vi "PXI-Create Channels.vi"(0 "Task Specification Array In":T1[](array[typedef]) {"Channels"."Terminal configuration" items=["Default"=-1, "RSE"=10083, "Differential"=10106, "Pseudodifferential"=12529]}, 11 "error in (no error)":errorcluster) -> (4 "Task Specification Array Out":T1[](array[typedef]) {"Channels"."Terminal configuration" items=["Default"=-1, "RSE"=10083, "Differential"=10106, "Pseudodifferential"=12529]}, 15 "error out":errorcluster)   [LabVIEW 2020]
uses:
  Type Defs/Task Specification Struct.ctl
  Type Defs/Channel Struct.ctl
  PXI Globals.vi
  <vilib>/DAQmx/create/channels.llb/DAQmx Create Channel (AI-Voltage-Basic).vi
  <vilib>/DAQmx/configure/timing.llb/DAQmx Timing (Sample Clock).vi
  <vilib>/DAQmx/create/channels.llb/DAQmx Create Channel (AO-Voltage-Basic).vi
  <resource>/objmgr/daqmx.rc
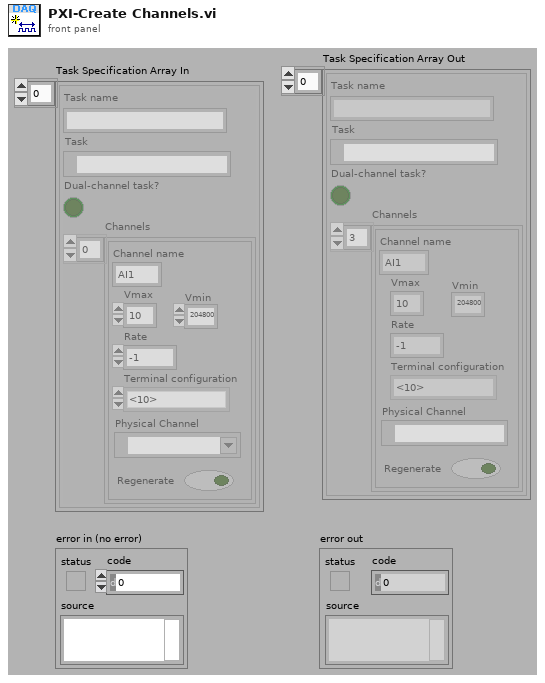
[diagram p1: front panel]
types:
  T1 = typedef "Task Specification Struct.ctl" = cluster{"Task name":string, "Task":refnum<k21>, "Dual-channel task?":bool, "Channels":T2[]}
  T2 = typedef "Channel Struct.ctl" = cluster{"Channel name":string, "Vmax":dbl, "Vmin":dbl, "Rate":dbl, "Terminal configuration":i32, "Physical Channel":tag, "Regenerate":bool}
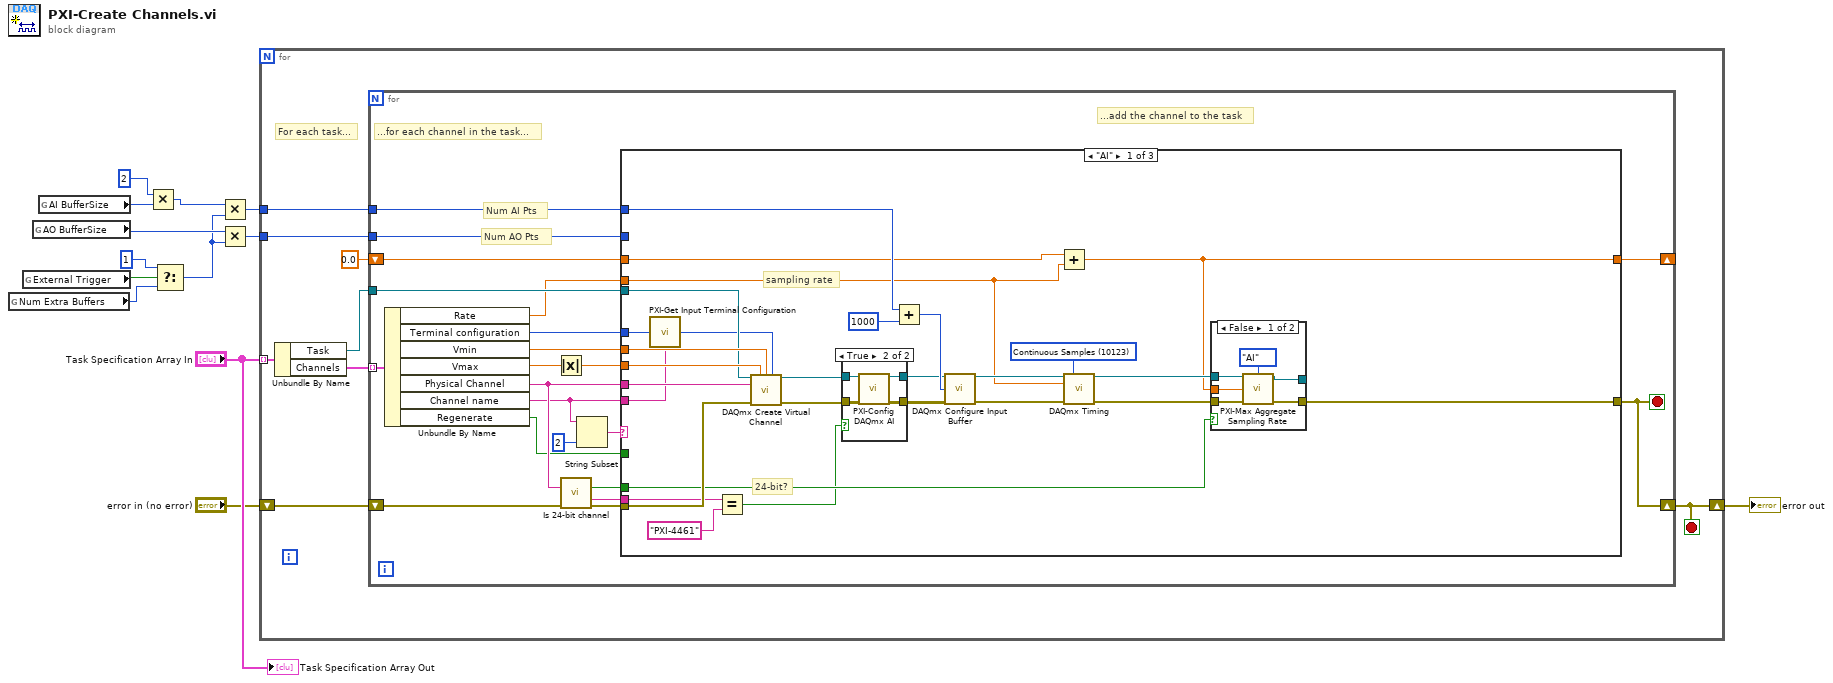
[diagram p0: block diagram]
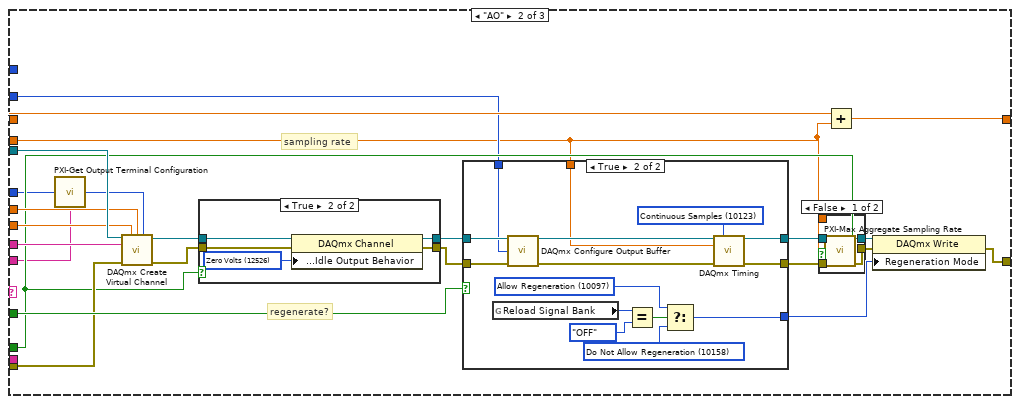
[diagram p4: hidden frame]
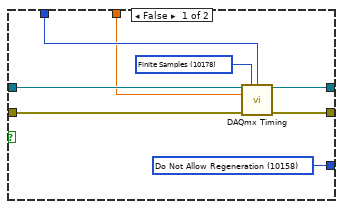
[diagram p6: hidden frame]
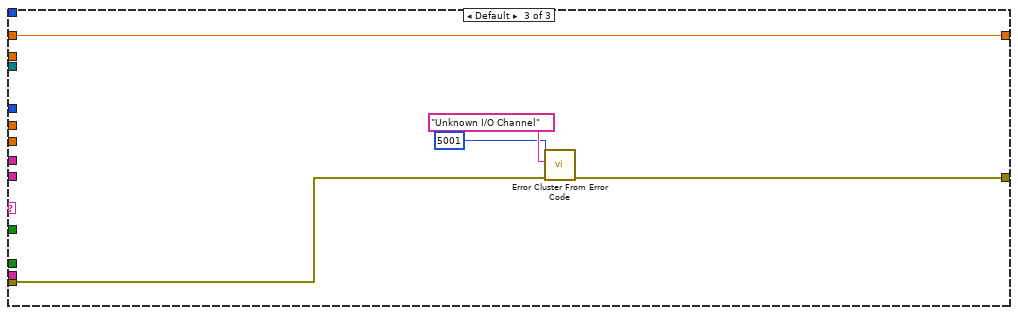
[diagram p8: hidden frame]
diagram:
  n1 = global read "PXI Globals.vi" "Num Extra Buffers"() -> (w5:i32)
  n2 = global read "PXI Globals.vi" "External Trigger"() -> (w7:bool)
  n3 = global read "PXI Globals.vi" "AO BufferSize"() -> (w12:i32)
  n4 = global read "PXI Globals.vi" "AI BufferSize"() -> (w13:i32)
  n5 = Multiply(x=2, y=w13) -> (x*y=w9:i32)
  n6 = Select(t=1, s=w7, f=w5) -> (s? t:f=w6:i32)
  n7 = Multiply(x=w9, y=w6) -> (x*y=w10:i32)
  n8 = Multiply(x=w12, y=w6) -> (x*y=w11:i32)
  n9 = for {
    tunnel: "Task Specification Array In" -> [w20] mode=indexing
    tunnel: w11 -> [w19]
    tunnel: w10 -> [w18]
    shift-right: [w14] -> w1
    shift-left: "error in (no error)" -> [w15]
    stop <- w14 stop-if-true
    # "For each task..."
    n10 = Unbundle By Name(w20) -> ("Task"=w16:refnum<k21>, "Channels"=w21:T2[])
    n11 = for {
      tunnel: w21 -> [w40] mode=indexing
      shift-right: [w23] -> w14
      shift-left: w15 -> [w33]
      tunnel: w16 -> [w39]
      tunnel: w19 -> [w28]
      tunnel: w18 -> [w27]
      shift-right: [w25] -> _
      shift-left: 0.0 -> [w26]
      stop <- w23 stop-if-true
      # "Num AI Pts"
      # "Num AO Pts"
      # "...add the channel to the task"
      # "...for each channel in the task..."
      n12 = Unbundle By Name(w40) -> ("Rate"=w38:dbl, "Terminal configuration"=w30:i32, "Vmin"=w36:dbl, "Vmax"=w35:dbl, "Physical Channel"=w34:tag, "Channel name"=w22:string, "Regenerate"=w31:bool)
      n13 = Absolute Value(x=w35) -> (abs(x)=w37:dbl)
      n14 = call "Is 24-bit channel.vi"("DAQmx Physical Channel"=w34, "error in (no error)"=w33) -> ("is 24bit?"=w29:bool, "ProductType"=w24:string, "error out"=w32:errorcluster)  [unwired: 11 in]
      n15 = String Subset(string=w22, length (rest)=2 ("length (rest)")) -> (substring=w41:string)  [unwired: 1 in]
      n16 = case shown="\"AI\"" w41 {
        tunnel: w34 -> [w70 w107 _]
        tunnel: w36 -> [w69 w103 _]
        tunnel: w37 -> [w68 w104 _]
        tunnel: w32 -> [w67 w105 w148]
        tunnel: [w50 w98 w147] -> w23
        tunnel: w39 -> [w66 w106 _]
        tunnel: w38 -> [w55 w89 _]
        tunnel: w31 -> [_ w108 _]
        tunnel: w30 -> [w45 w88 _]
        tunnel: w29 -> [w51 w93 _]
        tunnel: w28 -> [_ w92 _]
        tunnel: w27 -> [w57 _ _]
        tunnel: w26 -> [w56 w97 w146]
        tunnel: [w52 w96 w146] -> w25
        tunnel: w24 -> [w48 _ _]
        tunnel: w22 -> [w44 w85 _]
        frame "AI" {
          w58 = 10123 items=["Finite Samples"=10178, "Continuous Samples"=10123, "Hardware Timed Single Point"=12522] ("sample mode")
          # "24-bit?"
          # "sampling rate"
          n17 = call "PXI-Get Input Terminal Configuration.vi"("term config in"=w45, "channel"=w44) -> ("term config out"=w43:i32)  [unwired: 12 in, 1 out]
          n18 = Equal?(x=w48, y="PXI-4461") -> (x = y?=w46:bool)
          n19 = call-poly <vilib>:"DAQmx Create Virtual Channel.vi"("task in"=w66, "maximum value"=w68, "minimum value"=w69, "input terminal configuration"=w43, "physical channels"=w70, "error in"=w67) -> ("task out"=w61:refnum<k21>, "error out"=w60:errorcluster)  [unwired: 8 in]
          n20 = case shown="True" w46 {
            tunnel: w61 -> [w79 w84]
            tunnel: w60 -> [w80 w83]
            tunnel: [w80 w82] -> w59
            tunnel: [w79 w81] -> w49
            frame False {
            }
            frame True {
              n21 = call "PXI-Config DAQmx AI.vi"("task in"=w84, "error in"=w83) -> ("task out"=w81:refnum<k21>, "error out"=w82:errorcluster)  [unwired: 12 in]
            }
          }
          n22 = Add(x=w57, y=1000) -> (x+y=w62:i32)
          n23 = call <vilib>:"DAQmx Configure Input Buffer.vi"("task/channels in"=w49, "buffer size (in samples per channel)"=w62, "error in"=w59) -> ("task out"=w65:refnum<k21>, "error out"=w64:errorcluster)  [unwired: 11 in]
          n24 = Add(x=w56, y=w55) -> (x+y=w52:dbl)
          n25 = call-poly <vilib>:"DAQmx Timing.vi"("task/channels in"=w65, "sample mode"=w58, "rate"=w55, "error in"=w64) -> ("task out"=w53:refnum<k21>, "error out"=w54:errorcluster)  [unwired: 10 in]
          n26 = case shown="False" w51 {
            tunnel: w54 -> [w76 w77]
            tunnel: w53 -> [w75 w78]
            tunnel: [w74 w77] -> w50
            tunnel: [w73 w78] -> _
            tunnel: w52 -> [w72 _]
            frame False {
              n27 = call "PXI-Max Aggregate Sampling Rate.vi"("task in"=w75, "Mode"=enum16{"AO", "AI", "DO", "DI"}."AI", "Agg Sampling Rate"=w72, "error in (no error)"=w76) -> ("task out"=w73:refnum<k21>, "error out"=w74:errorcluster)  [unwired: 9 in, 1 out]
            }
            frame True {
            }
          }
        }
        frame "AO" {
          # "sampling rate"
          # "regenerate?"
          n28 = call "PXI-Get Output Terminal Configuration.vi"("term config in"=w88, "key"=w85) -> ("term config out"=w86:i32)  [unwired: 12 in, 1 out]
          n29 = call-poly <vilib>:"DAQmx Create Virtual Channel.vi"("task in"=w106, "maximum value"=w104, "minimum value"=w103, "output terminal configuration"=w86, "physical channels"=w107, "error in"=w105) -> ("task out"=w87:refnum<k21>, "error out"=w102:errorcluster)  [unwired: 8 in]
          n30 = case shown="True" w93 {
            tunnel: [w110 w115] -> w101
            tunnel: [w109 w114] -> w100
            tunnel: w87 -> [w110 w112]
            tunnel: w102 -> [w109 w111]
            frame False {
            }
            frame True {
              w113 = 12526 items=["Zero Volts"=12526, "High Impedance"=12527, "Maintain Existing Value"=12528] ("AO.IdleOutputBehavior")
              n31 = property class="DAQmx Channel"(reference=w112, error in=w111, "Analog Output:General Properties:Output Configuration:Idle Output Behavior"=w113) -> (reference out=w115:refnum<k21>, error out=w114:errorcluster)
            }
          }
          n32 = case shown="True" w108 {
            tunnel: w101 -> [w122 w136]
            tunnel: w100 -> [w121 w135]
            tunnel: [w119 w126] -> w91
            tunnel: [w120 w127] -> w90
            tunnel: [w123 w131] -> w99
            tunnel: w92 -> [w117 w130]
            tunnel: w89 -> [w116 w124]
            frame False {
              w118 = 10178 items=["Finite Samples"=10178, "Continuous Samples"=10123, "Hardware Timed Single Point"=12522] ("sample mode")
              w123 = 10158 items=["Allow Regeneration"=10097, "Do Not Allow Regeneration"=10158] ("RegenMode")
              n33 = call-poly <vilib>:"DAQmx Timing.vi"("task/channels in"=w122, "sample mode"=w118, "samples per channel"=w117, "rate"=w116, "error in"=w121) -> ("task out"=w119:refnum<k21>, "error out"=w120:errorcluster)  [unwired: 9 in]
            }
            frame True {
              w133 = 10097 items=["Allow Regeneration"=10097, "Do Not Allow Regeneration"=10158] ("RegenMode")
              w132 = 10158 items=["Allow Regeneration"=10097, "Do Not Allow Regeneration"=10158] ("RegenMode")
              w125 = 10123 items=["Finite Samples"=10178, "Continuous Samples"=10123, "Hardware Timed Single Point"=12522] ("sample mode")
              n34 = global read "PXI Globals.vi" "Reload Signal Bank"() -> (w138:enum32{"OFF", "ENABLED", "FORCED"})
              n35 = call <vilib>:"DAQmx Configure Output Buffer.vi"("task/channels in"=w136, "buffer size (in samples per channel)"=w130, "error in"=w135) -> ("task out"=w129:refnum<k21>, "error out"=w128:errorcluster)  [unwired: 11 in]
              n36 = Equal?(x=w138, y=enum16{"OFF", "ENABLED", "FORCED"}."OFF") -> (x = y?=w134:bool)
              n37 = Select(t=w133, s=w134, f=w132) -> (s? t:f=w131:i32)
              n38 = call-poly <vilib>:"DAQmx Timing.vi"("task/channels in"=w129, "sample mode"=w125, "rate"=w124, "error in"=w128) -> ("task out"=w126:refnum<k21>, "error out"=w127:errorcluster)  [unwired: 10 in]
            }
          }
          n39 = case shown="False" w93 {
            tunnel: w90 -> [w143 w144]
            tunnel: [w142 w144] -> w95
            tunnel: w91 -> [w141 w145]
            tunnel: [w140 w145] -> w94
            tunnel: w89 -> [w139 _]
            frame False {
              n40 = call "PXI-Max Aggregate Sampling Rate.vi"("task in"=w141, "Agg Sampling Rate"=w139, "error in (no error)"=w143) -> ("task out"=w140:refnum<k21>, "error out"=w142:errorcluster)  [unwired: 10 in, 1 out]
            }
            frame True {
            }
          }
          n41 = Add(x=w97, y=w89) -> (x+y=w96:dbl)
          n42 = property class="DAQmx Write"(reference=w94, error in=w95, "Regeneration Mode"=w99) -> (error out=w98:errorcluster)  [unwired: 1 out]
        }
        frame Default {
          n43 = call <vilib>:"Error Cluster From Error Code.vi"("error in (no error)"=w148, "error message (\"\")"="Unknown I/O Channel" ("error message (\"\")"), "error code (0)"=5001) -> ("error out"=w147:errorcluster)  [unwired: 6 in]
        }
      }
    }
  }
  "error out" <- w1
  "Task Specification Array Out" <- "Task Specification Array In"
